vi "qp_parameter check.vi"(7 "X0":dbl[](array[numeric]), 8 "error in (no error)":errorcluster, 11 "qp data in":T1) -> (0 "error out":errorcluster, 3 "qp data in":T1)   [LabVIEW 2018, in "NI_Gmath.lvlib"]
uses:
  NI_Gmath.lvlib
  qp_problem data.ctl
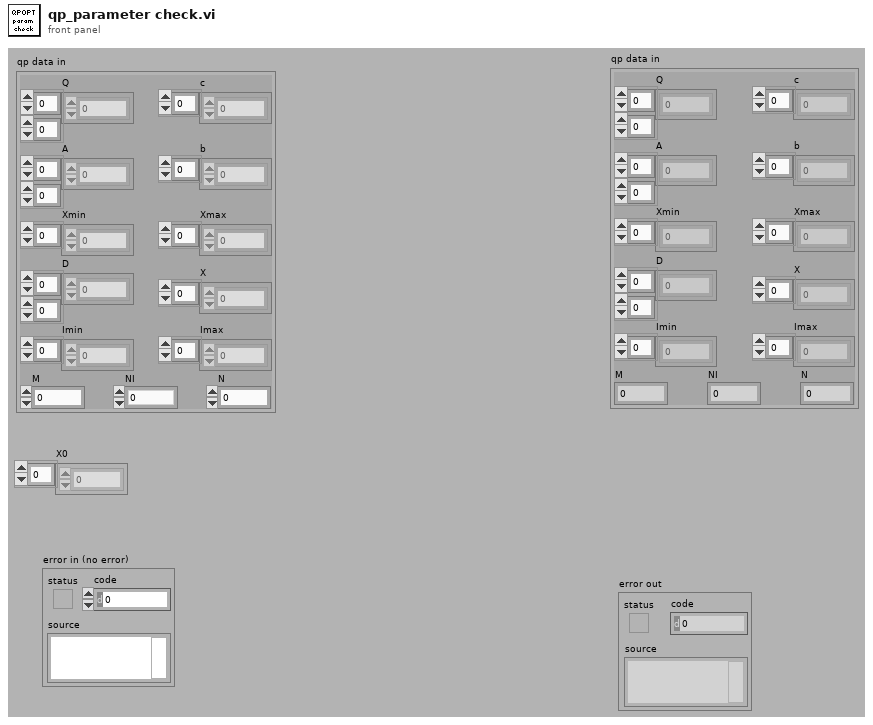
[diagram p1: front panel]
types:
  T1 = typedef "NI_Gmath.lvlib/qp_problem data.ctl" = cluster{"Q":dbl[][], "c":dbl[], "A":dbl[][], "b":dbl[], "Xmin":dbl[], "Xmax":dbl[], "M":i32, "N":i32, "D":dbl[][], "Imax":dbl[], "Imin":dbl[], "NI":i32, "X":dbl[]}
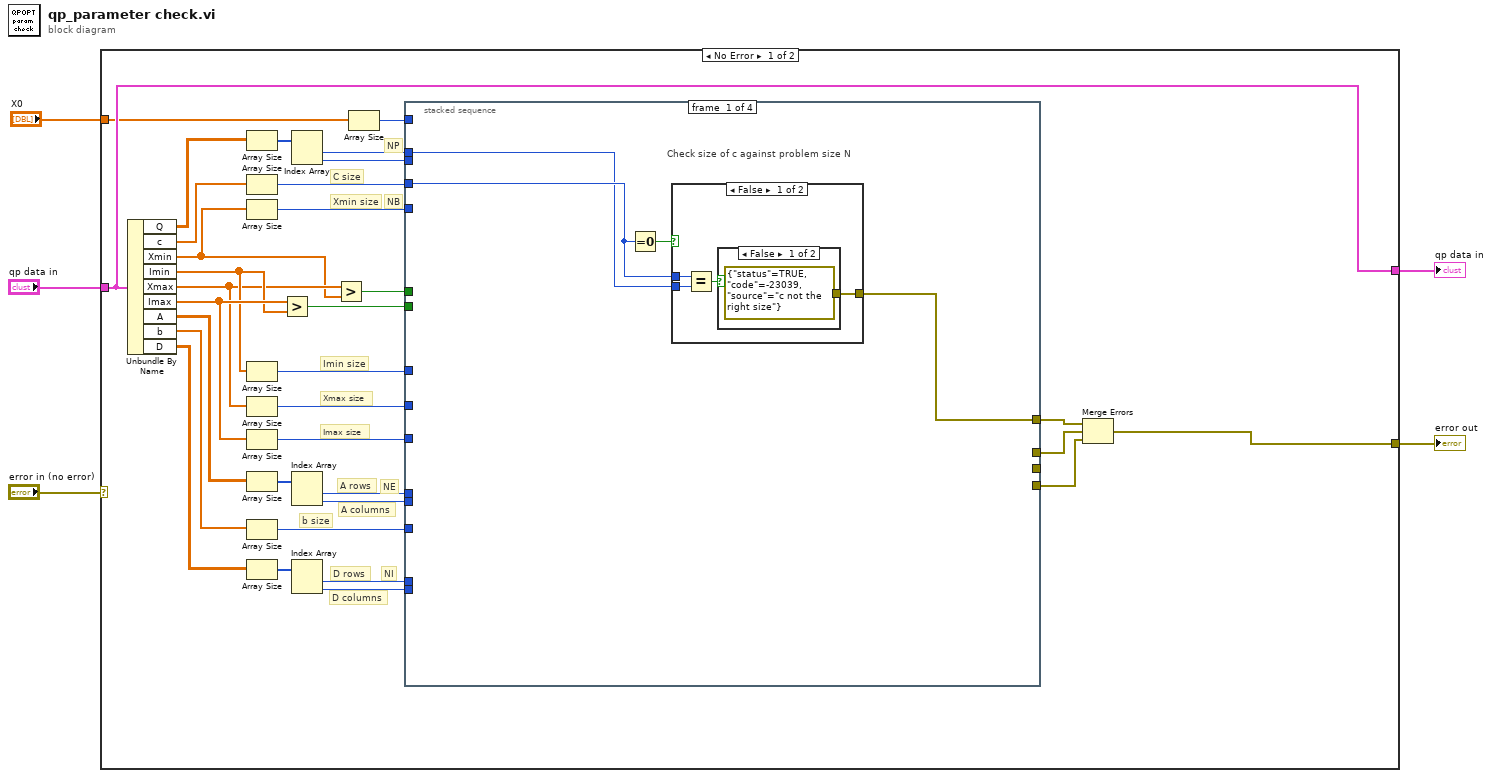
[diagram p0: block diagram]
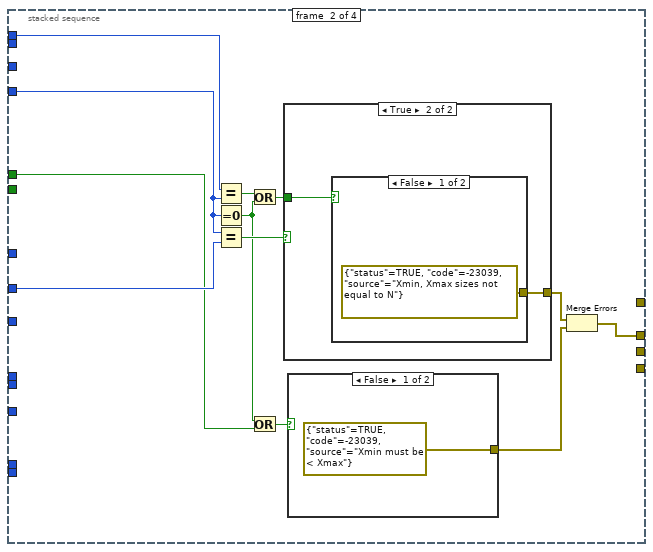
[diagram p4: hidden frame]
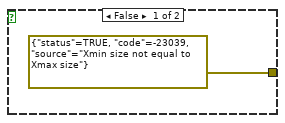
[diagram p6: hidden frame]
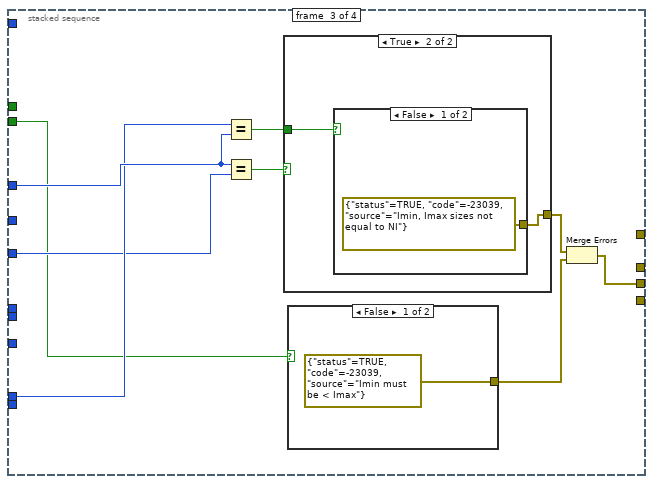
[diagram p8: hidden frame]
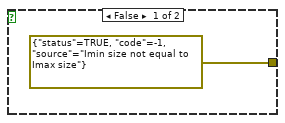
[diagram p10: hidden frame]
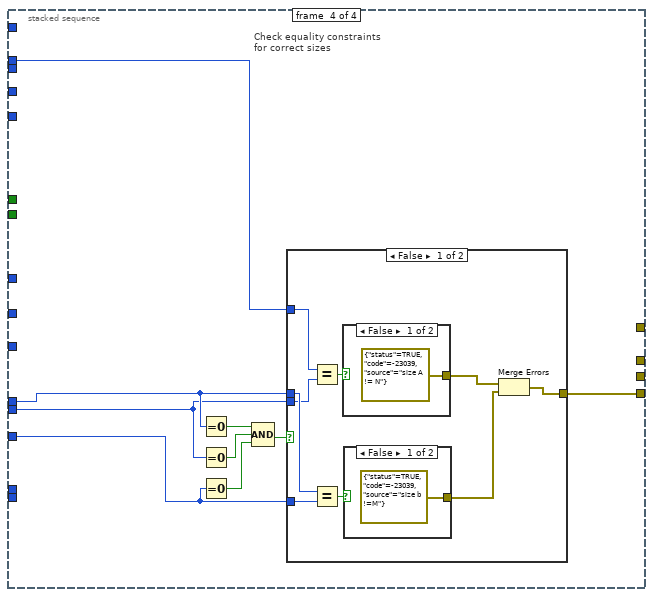
[diagram p12: hidden frame]
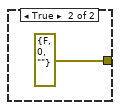
[diagram p13: hidden frame]
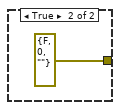
[diagram p14: hidden frame]
diagram:
  n1 = case shown="No Error" "error in (no error)" {
    selector: "error in (no error)" -> [_ w102]
    tunnel: [w36 w102] -> w2
    tunnel: "qp data in" -> [w14 w101]
    tunnel: [w14 w101] -> w3
    tunnel: "X0" -> [w13 _]
    frame No Error {
      # "NI"
      # "NE"
      # "NB"
      # "NP"
      # "C size"
      # "D columns"
      # "D rows"
      # "b size"
      # "A columns"
      # "A rows"
      # "Imax size"
      # "Xmax size"
      # "Imin size"
      # "Xmin size"
      n2 = Unbundle By Name(w14) -> ("Q"=w31:dbl[][], "c"=w29:dbl[], "Xmin"=w7:dbl[], "Imin"=w10:dbl[], "Xmax"=w8:dbl[], "Imax"=w11:dbl[], "A"=w27:dbl[][], "b"=w26:dbl[], "D"=w25:dbl[][])
      n3 = Array Size(array=w31) -> (size(s)=w34:i32[])
      n4 = Array Size(array=w29) -> (size(s)=w30:i32)
      n5 = Array Size(array=w7) -> (size(s)=w28:i32)
      n6 = Array Size(array=w10) -> (size(s)=w22:i32)
      n7 = Array Size(array=w8) -> (size(s)=w21:i32)
      n8 = Array Size(array=w11) -> (size(s)=w20:i32)
      n9 = Array Size(array=w27) -> (size(s)=w23:i32[])
      n10 = Array Size(array=w26) -> (size(s)=w17:i32)
      n11 = Array Size(array=w25) -> (size(s)=w24:i32[])
      n12 = Greater?(x=w11, y=w10) -> (0:w9:bool)
      n13 = Index Array(array=w34) -> (element #1=w33:i32, element #2=w32:i32)  [unwired: 2 in]
      n14 = Index Array(array=w23) -> (element #1=w19:i32, element #2=w18:i32)  [unwired: 2 in]
      n15 = Index Array(array=w24) -> (element #1=w16:i32, element #2=w15:i32)  [unwired: 2 in]
      n16 = Greater?(x=w8, y=w7) -> (0:w6:bool)
      n17 = Array Size(array=w13) -> (size(s)=w12:i32)
      n18 = stacked-sequence {
        tunnel: [w41 _ _ _] -> w38
        tunnel: [_ w56 _ _] -> w37
        tunnel: [_ _ _ w87] -> w35
        tunnel: [_ _ w69 _] -> _
        tunnel: w33 -> [w39 w49 _ w79]
        tunnel: w32 -> [_ _ _ _]
        tunnel: w30 -> [w40 _ _ _]
        tunnel: w28 -> [_ w51 _ _]
        tunnel: w22 -> [_ _ w68 _]
        tunnel: w21 -> [_ w50 _ _]
        tunnel: w20 -> [_ _ w66 _]
        tunnel: w19 -> [_ _ _ w82]
        tunnel: w18 -> [_ _ _ w81]
        tunnel: w17 -> [_ _ _ w80]
        tunnel: w16 -> [_ _ w67 _]
        tunnel: w15 -> [_ _ _ _]
        tunnel: w12 -> [_ _ _ _]
        tunnel: w9 -> [_ _ w65 _]
        tunnel: w6 -> [_ w48 _ _]
        frame #0 {
          # "Check size of c against problem size N"
          n19 = Equal To 0?(x=w40) -> (x = 0?=w42:bool)
          n20 = case shown="False" w42 {
            tunnel: w39 -> [w43 _]
            tunnel: w40 -> [w44 _]
            tunnel: [w45 _] -> w41
            frame False {
              n21 = Equal?(x=w44, y=w43) -> (x = y?=w46:bool)
              n22 = case shown="False" w46 {
                tunnel: [errorcluster {"status"=TRUE, "code"=-23039, "source"="c not the right size"} ("error in (no error)") _] -> w45
                frame False {
                }
                frame True {
                }
              }
            }
            frame True {
            }
          }
        }
        frame #1 {
          n23 = Equal?(x=w49, y=w51) -> (x = y?=w55:bool)
          n24 = Equal To 0?(x=w51) -> (x = 0?=w53:bool)
          n25 = Equal?(x=w51, y=w50) -> (x = y?=w59:bool)
          n26 = Or(x=w55, y=w53) -> (x .or. y?=w54:bool)
          n27 = Or(x=w53, y=w48) -> (x .or. y?=w52:bool)
          n28 = case shown="True" w59 {
            tunnel: [errorcluster {"status"=TRUE, "code"=-23039, "source"="Xmin size not equal to Xmax size"} ("error in (no error)") w63] -> w58
            tunnel: w54 -> [_ w62]
            frame False {
            }
            frame True {
              n29 = case shown="False" w62 {
                tunnel: [errorcluster {"status"=TRUE, "code"=-23039, "source"="Xmin, Xmax sizes not equal to N"} ("error in (no error)") _] -> w63
                frame False {
                }
                frame True {
                }
              }
            }
          }
          n30 = case shown="False" w52 {
            tunnel: [errorcluster {"status"=TRUE, "code"=-23039, "source"="Xmin must be < Xmax"} ("error in (no error)") _] -> w57
            frame False {
            }
            frame True {
            }
          }
          n31 = Merge Errors(w58, w57) -> (w56:errorcluster)
        }
        frame #2 {
          n32 = Equal?(x=w67, y=w68) -> (x = y?=w70:bool)
          n33 = Equal?(x=w68, y=w66) -> (x = y?=w73:bool)
          n34 = case shown="True" w73 {
            tunnel: [errorcluster {"status"=TRUE, "code"=-1, "source"="Imin size not equal to Imax size"} ("error in (no error)") w77] -> w72
            tunnel: w70 -> [_ w76]
            frame False {
            }
            frame True {
              n35 = case shown="False" w76 {
                tunnel: [errorcluster {"status"=TRUE, "code"=-23039, "source"="Imin, Imax sizes not equal to NI"} ("error in (no error)") _] -> w77
                frame False {
                }
                frame True {
                }
              }
            }
          }
          n36 = case shown="False" w65 {
            tunnel: [errorcluster {"status"=TRUE, "code"=-23039, "source"="Imin must be < Imax"} ("error in (no error)") _] -> w71
            frame False {
            }
            frame True {
            }
          }
          n37 = Merge Errors(w72, w71) -> (w69:errorcluster)
        }
        frame #3 {
          # "Check equality constraints\nfor correct sizes"
          n38 = Equal To 0?(x=w82) -> (x = 0?=w86:bool)
          n39 = Equal To 0?(x=w81) -> (x = 0?=w85:bool)
          n40 = Equal To 0?(x=w80) -> (x = 0?=w84:bool)
          n41 = Compound Arithmetic op=AND(w86, w85, w84) -> (w83:bool)
          n42 = case shown="False" w83 {
            tunnel: [w93 _] -> w87
            tunnel: w82 -> [w91 _]
            tunnel: w81 -> [w90 _]
            tunnel: w80 -> [w89 _]
            tunnel: w79 -> [w88 _]
            frame False {
              n43 = Equal?(x=w88, y=w90) -> (x = y?=w96:bool)
              n44 = Equal?(x=w91, y=w89) -> (x = y?=w95:bool)
              n45 = case shown="False" w96 {
                tunnel: [errorcluster {"status"=TRUE, "code"=-23039, "source"="size A != N"} ("error in (no error)") errorcluster {"status"=FALSE, "code"=0, "source"=""} ("error in (no error)")] -> w92
                frame False {
                }
                frame True {
                }
              }
              n46 = case shown="False" w95 {
                tunnel: [errorcluster {"status"=TRUE, "code"=-23039, "source"="size b !=M"} ("error in (no error)") errorcluster {"status"=FALSE, "code"=0, "source"=""} ("error in (no error)")] -> w94
                frame False {
                }
                frame True {
                }
              }
              n47 = Merge Errors(w92, w94) -> (w93:errorcluster)
            }
            frame True {
            }
          }
        }
      }
      n48 = Merge Errors(w38, w37, w35) -> (w36:errorcluster)
    }
    frame Error {
    }
  }
  "error out" <- w2
  "qp data in" <- w3
